vi "XLP80_CAN_SearchWrongName.vi"() -> ()   [LabVIEW 2021]
uses:
  <vilib>/nican/nicantsk.llb/CAN Interface.ctl
  XLP80_Globals/Globals_Settings_XLP80.vi
panel:
  out "Signal Name":string[](array[string])
  out "size(s)":i32
  out "first subarray":string[](array[string])
  out "error out":errorcluster
  out "second subarray":string[](array[string])
  in  "index":i32
  # "LV_A_71_nmt_function"
  # "LV_A_71_PSU_Mode_Control_On"
  # "LV_A_71_PSU_Mode_Precharge_On"
  # "LV_A_H42_KL15_ENABLE"
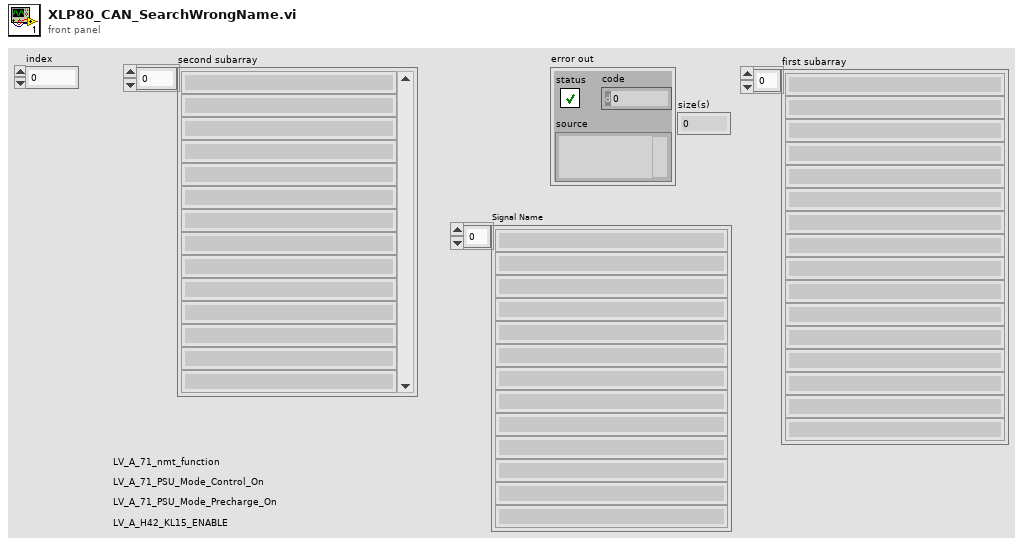
[diagram p1: front panel]
types:
  T1 = typedef "CAN Interface.ctl" = u16
  T2 = cluster{"Signal Name":string[], "Description":string[], "Unit":string[], "Min":dbl[], "Max":dbl[], "TestmodeA":bool[], "LogEnable":bool[]}
  T3 = typedef "CAN Task Reference.ctl" = u32
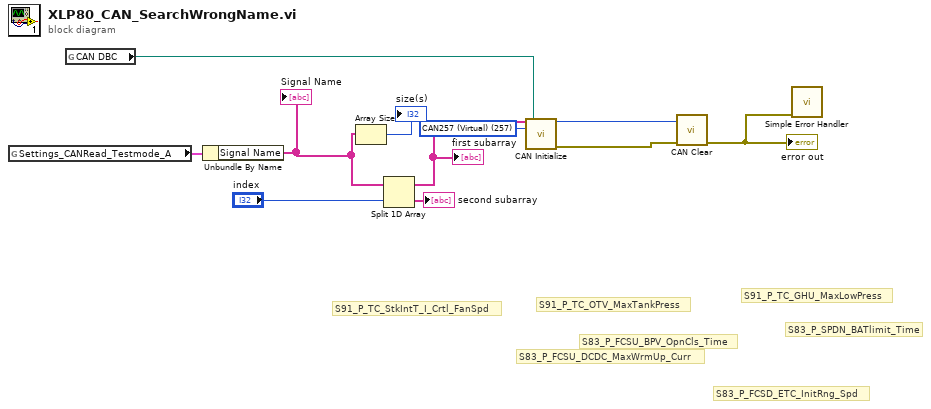
[diagram p0: block diagram]
diagram:
  w11 = T1 257 items=["CAN0"=0, "CAN1"=1, "CAN2"=2, "CAN3"=3, "CAN4"=4, "CAN5"=5, "CAN6"=6, "CAN7"=7, "CAN8"=8, "CAN9"=9, "CAN10"=10, "CAN11"=11, "CAN12"=12, "CAN13"=13, "CAN14"=14, "CAN15"=15, "CAN16"=16, "CAN17"=17, "CAN18"=18, "CAN19"=19, "CAN20"=20, "CAN21"=21, "CAN22"=22, "CAN23"=23, "CAN24"=24, "CAN25"=25, "CAN26"=26, "CAN27"=27, "CAN28"=28, "CAN29"=29, "CAN30"=30, "CAN31"=31, "CAN32"=32, "CAN33"=33, "CAN34"=34, "CAN35"=35, "CAN36"=36, "CAN37"=37, "CAN38"=38, "CAN39"=39, "CAN40"=40, "CAN41"=41, "CAN42"=42, "CAN43"=43, "CAN44"=44, "CAN45"=45, "CAN46"=46, "CAN47"=47, "CAN48"=48, "CAN49"=49, "CAN50"=50, "CAN51"=51, "CAN52"=52, "CAN53"=53, "CAN54"=54, "CAN55"=55, "CAN56"=56, "CAN57"=57, "CAN58"=58, "CAN59"=59, "CAN60"=60, "CAN61"=61, "CAN62"=62, "CAN63"=63, "MAX default"=64, "CAN256 (Virtual)"=256, "CAN257 (Virtual)"=257] ("interface")
  # "S91_P_TC_StkIntT_I_Crtl_FanSpd"
  # "S91_P_TC_OTV_MaxTankPress"
  # "S91_P_TC_GHU_MaxLowPress"
  # "S83_P_SPDN_BATlimit_Time"
  # "S83_P_FCSU_DCDC_MaxWrmUp_Curr"
  # "S83_P_FCSU_BPV_OpnCls_Time"
  # "S83_P_FCSD_ETC_InitRng_Spd"
  n1 = global read "Globals_Settings_XLP80.vi" "Settings_CANRead_Testmode_A"() -> (w2:T2)
  n2 = global read "Globals_Settings_XLP80.vi" "CAN DBC"() -> (w10:path)
  n3 = Unbundle By Name(w2) -> ("Signal Name"=w1:string[])
  "Signal Name" <- w1
  n4 = Array Size(array=w1) -> (size(s)=→"size(s)":i32)
  n5 = Split 1D Array(array=w1, index="index") -> (first subarray=w6:string[], second subarray=→"second subarray":string[])
  "first subarray" <- w6
  n6 = call <vilib>:"CAN Initialize.vi"("channel list"=w6, "filepath"=w10, "interface"=w11) -> ("task reference out"=w8:T3, "error out"=w9:errorcluster)  [unwired: 11 in]
  n7 = call <vilib>:"CAN Clear.vi"("error in (no error)"=w9, "task reference in"=w8) -> ("error out"=w4:errorcluster)  [unwired: 9 in]
  "error out" <- w4
  n8 = call <vilib>:"Simple Error Handler.vi"("error in (no error)"=w4) -> ()  [unwired: 4 in, 5 out]
